vi "Blink.vi"(9 "String":string, 10 "Acessors:Running":bool, 11 "Checkbox":bool) -> (3 "f":string)   [LabVIEW 2025, in "DAQ_Module.lvlib" / "DAQ_Module.lvclass"]
uses:
  DAQ_Module.lvclass
  DAQ_Module.lvclass/DAQ_Module.ctl
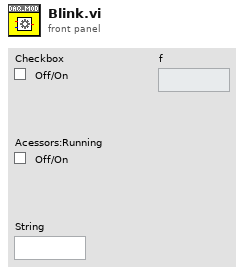
[diagram p1: front panel]
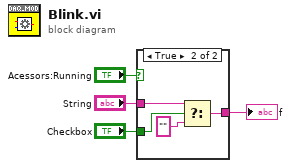
[diagram p0: block diagram]
diagram:
  n1 = case shown="True" "Acessors:Running" {
    tunnel: "String" -> [w5 w9]
    tunnel: [w5 w7] -> w2
    tunnel: "Checkbox" -> [_ w6]
    frame False {
    }
    frame True {
      n2 = Select(t=w9, s=w6, f="") -> (s? t:f=w7:string)
    }
  }
  "f" <- w2
